vi "PUT Graph Data.vi"(0 "Graph Data":cluster{"X":dbl[], "Y":dbl[]}) -> ()   [LabVIEW 2013]
uses:
  Action.ctl
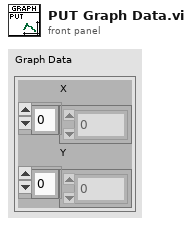
[diagram p1: front panel]
types:
  T1 = typedef "Action.ctl" = enum16{"GET", "PUT", "DELETE"}
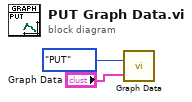
[diagram p0: block diagram]
diagram:
  n1 = call "Graph Data.vi"("Input"="Graph Data", "Action"=Action."PUT") -> ()  [unwired: 1 in, 1 out]
